vi "SUB-Data conv_INT to double.vi"(3 "U32":u32 format="%x") -> (1 "FP32":sgl format="%.10f")   [LabVIEW 2015]
panel:
  # "데이터 변환 : 24비트 데이터를 부호없는고정소수로 변환 (3비트 정수 + 21비트 분수)"
  # "Unsigned fixed-point number\n    3 bits integer\n  21 bits fractional"
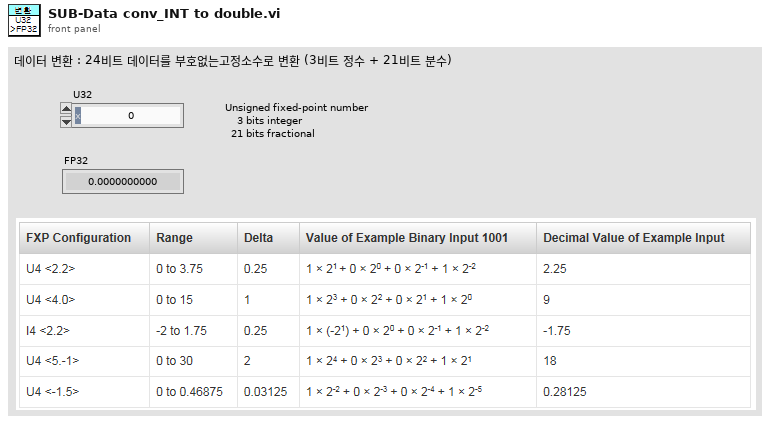
[diagram p1: front panel]
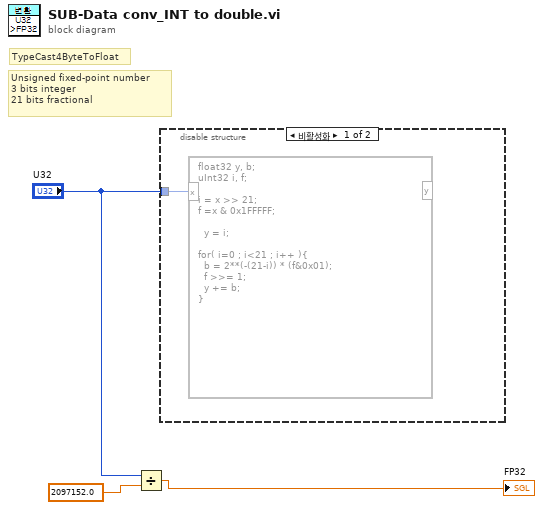
[diagram p0: block diagram]
diagram:
  # "Unsigned fixed-point number\n3 bits integer\n21 bits fractional"
  # "TypeCast4ByteToFloat"
  n1 = Divide(x="U32", y=sgl 2097152.0) -> (x/y=→"FP32":sgl)
  n2 = disable-structure shown="비활성화" {
    disable-tunnel: "U32" -> [w4 _]
    frame Disabled {
      n3 = formula code="float32 y, b;\nuInt32 i, f;\n\ni = x >> 21;\nf =x & 0x1FFFFF;\n\n  y = i;\n\nfor( i=0 ; i<21 ; i++ ){\n  b = 2**(-(21-i)) * (f&0x01);\n  f >>= 1;\n  y += b;\n}"("x"=w4) -> ()  [unwired: 1 out]
    }
    frame Enabled {
    }
  }
